vi "_ConvertOneParameter.vi"(2 "Parameter":string[](array[string]), 3 "LensTableIn":T1[](array[typedef])) -> (0 "Found":bool, 1 "LensTableOut":T1[](array[typedef]))   [LabVIEW 2015]
uses:
  Type/_Lens Property.ctl
  Type/_Log Command.ctl
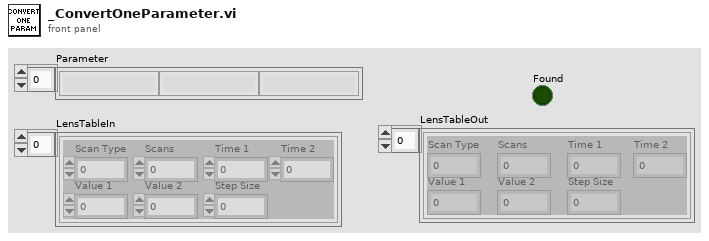
[diagram p1: front panel]
types:
  T1 = typedef "_Lens Property.ctl" = cluster{"Scan Type":u8, "Scans":i32, "Time 1":dbl, "Time 2":dbl, "Value 1":dbl, "Value 2":dbl, "Step Size":dbl}
  T2 = typedef "_Log Command.ctl" = enum16{"No Command", "Open", "Read", "Write", "Close", "Check Size"}
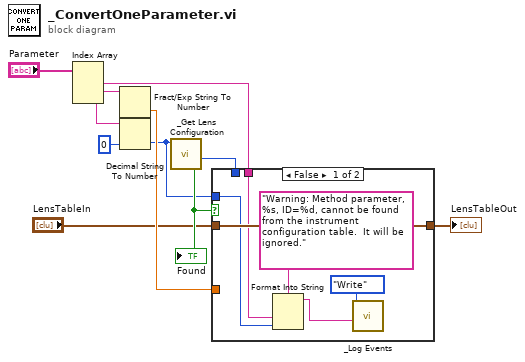
[diagram p0: block diagram]
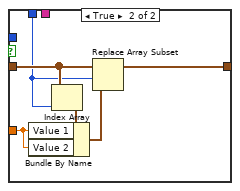
[diagram p2: hidden frame]
diagram:
  n1 = Index Array(array="Parameter") -> (element #1=w2:string, element #2=w3:string, element #3=w4:string)  [unwired: 3 in]
  n2 = Fract/Exp String To Number(string=w3) -> (number=w10:dbl)  [unwired: 3 in, 1 out]
  n3 = Decimal String To Number(string=w4, default (0L)=u8 0 ("default (0 I32)")) -> (number=w1:u8)  [unwired: 1 in, 1 out]
  n4 = call "_Get Lens Configuration.vi"("Channel #"=w1) -> ("Found"=w11:bool, "Config Row#"=w9:i32)  [unwired: 1 in, 4 out]
  "Found" <- w11
  n5 = case shown="False" w11 {
    tunnel: [w17 w21] -> w7
    tunnel: "LensTableIn" -> [w17 w20]
    tunnel: w9 -> [_ w19]
    tunnel: w10 -> [_ w18]
    tunnel: w2 -> [w16 _]
    tunnel: w1 -> [w15 _]
    frame False {
      n6 = Format Into String(format string="Warning: Method parameter, %s, ID=%d, cannot be found from the instrument configuration table.  It will be ignored.", w16, w15) -> (resulting string=w13:string)  [unwired: 2 in, 1 out]
      n7 = call "_Log Events.vi"("Event"=w13, "Log Command"=_Log_Command."Write") -> ()  [unwired: 6 in, 2 out]
    }
    frame True {
      n8 = Index Array(array=w20, index=w19) -> (element=w23:T1)
      n9 = Bundle By Name(cluster=w23, "Value 1"=w18, "Value 2"=w18) -> (w22:T1)
      n10 = Replace Array Subset(array=w20, new element=w22, index=w19) -> (w21:T1[])
    }
  }
  "LensTableOut" <- w7
